vi "PV build_protocol.vi"(4 "Data":string="=?", 5 "Parameter-number":u16=309 max=999 step=1, 6 "parameter\nread<->describe":bool, 7 "Adress":u16=1 max=999 step=1) -> (0 "output":string="1230030902=?112\r")   [LabVIEW 2015, in "Pfeiffer Vacuum.lvlib"]
uses:
  Pfeiffer Vacuum.lvlib
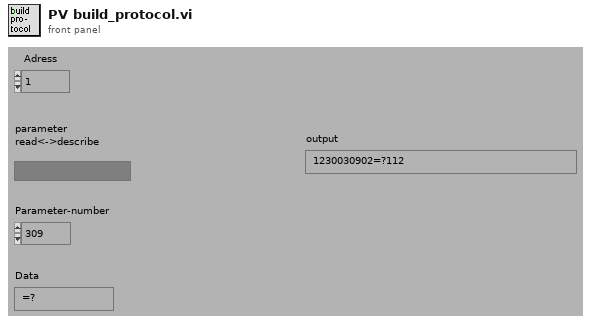
[diagram p1: front panel]
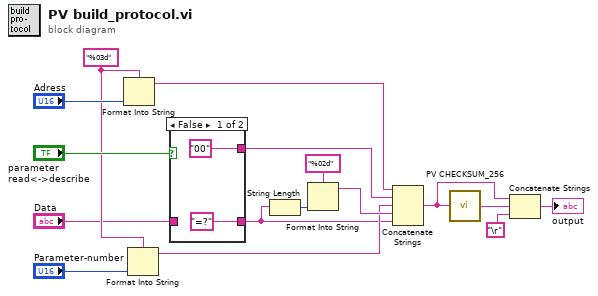
[diagram p0: block diagram]
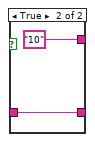
[diagram p2: hidden frame]
diagram:
  w6 = "%03d" ("Format-String")
  n1 = Format Into String(format string=w6, "Adress") -> (resulting string=w10:string)  [unwired: 2 in, 1 out]
  n2 = Format Into String(format string=w6, "Parameter-number") -> (resulting string=w12:string)  [unwired: 2 in, 1 out]
  n3 = case shown="False" "parameter\nread<->describe" {
    tunnel: ["00" "10"] -> w8
    tunnel: "Data" -> [_ w19]
    tunnel: ["=?" w19] -> w1
    frame False {
    }
    frame True {
    }
  }
  n4 = String Length(string=w1) -> (length=w16:i32)
  n5 = Format Into String(format string="%02d" ("Format-String"), w16) -> (resulting string=w14:string)  [unwired: 2 in, 1 out]
  n6 = Concatenate Strings(w10, w8, w12, w14, w1) -> (w4:string)
  n7 = call "PV CHECKSUM_256.VI"("input string"=w4) -> ("checksum"=w3:string)
  n8 = Concatenate Strings(w4, w3, "\r") -> (→"output":string)
